vi "Coord window-Initialisation.vi"(6 "Force-clear Listbox":bool, 9 "Coordinate list window refs":T1, 11 "Disable window positioning":bool) -> (0 "error out":errorcluster, 2 "Window size":cluster{"Horisontal":i16, "Vertical":i16}, 3 "VI out":refnum<vi>)   [LabVIEW 2013]
uses:
  Typedefs/Coordinate list window refs.ctl
  Visualisation/Functional Imaging Viewer/SubVIs/Experiment header interface/Typedefs/Save-Load-Save as-Load last enum.ctl
  Globals/Coord window-Globals.vi
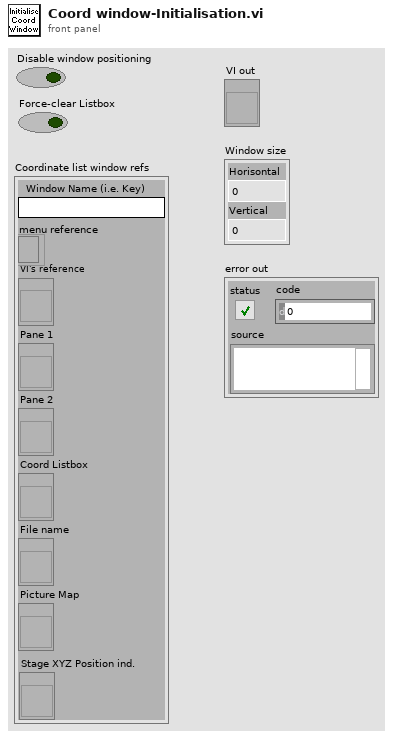
[diagram p1: front panel]
types:
  T1 = typedef "Coordinate list window refs.ctl" = cluster{"Window Name (i.e. Key)":string, "menu reference":refnum<k9>, "VI's reference":refnum<vi>, "Pane 1":refnum<vi>, "Pane 2":refnum<vi>, "Coord Listbox":refnum<vi>, "File name":refnum<vi>, "Picture Map":refnum<vi>, "Stage XYZ Position ind.":refnum<vi>}
  T2 = typedef "Save-Load-Save as-Load last enum.ctl" = enum16{"Save file", "Save file as", "Load file", "Load last file"}
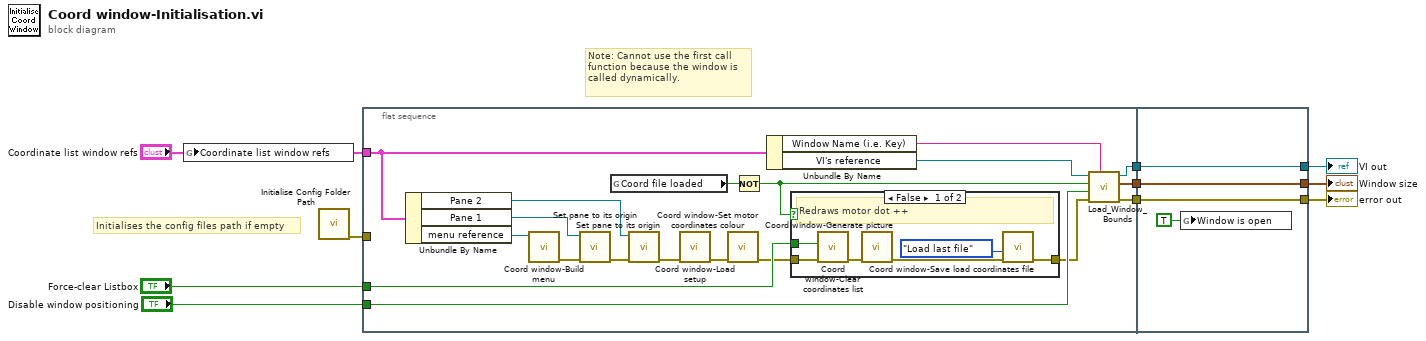
[diagram p0: block diagram]
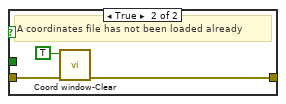
[diagram p2: hidden frame]
diagram:
  # "Initialises the config files path if empty"
  # "Note: Cannot use the first call function because the window is called dynamically."
  n1 = global write "Coord window-Globals.vi" "Coordinate list window refs"("Coordinate list window refs") -> ()
  n2 = call "Initialise Config Folder Path.vi"() -> ("error out"=w1:errorcluster)  [unwired: 9 in, 2 out]
  n3 = flat-sequence {
    tunnel: "Disable window positioning" -> [w24]
    tunnel: "Coordinate list window refs" -> [w19]
    tunnel: [w29] -> w5
    tunnel: [w23] -> w4
    tunnel: [w21] -> w3
    tunnel: "Force-clear Listbox" -> [w15]
    tunnel: w1 -> [_]
    tunnel: [w40] -> w7
    tunnel: [w41] -> w8
    tunnel: [w42] -> w10
    tunnel: w5 -> [w42]
    tunnel: w4 -> [w41]
    tunnel: w3 -> [w40]
    frame #0 {
      n4 = Unbundle By Name(w19) -> ("Pane 2"=w28:refnum<vi>, "Pane 1"=w27:refnum<vi>, "menu reference"=w26:refnum<k9>)
      n5 = call "Coord window-Build menu.vi"("menu"=w26) -> ("error out"=w25:errorcluster)  [unwired: 9 in, 1 out]
      n6 = call "Set pane to its origin.vi"("error in (no error)"=w25, "Pane Reference"=w27) -> ("error out (no error)"=w22:errorcluster)  [unwired: 8 in, 1 out]
      n7 = global read "Coord window-Globals.vi" "Coord file loaded"() -> (w17:bool)
      n8 = call "Set pane to its origin.vi"("error in (no error)"=w22, "Pane Reference"=w28) -> ("error out (no error)"=w14:errorcluster)  [unwired: 8 in, 1 out]
      n9 = call "Coord window-Load setup.vi"("error in (no error)"=w14) -> ("error out"=w13:errorcluster)  [unwired: 10 in]
      n10 = call "Coord window-Set motor coordinates colour.vi"("error in (no error)"=w13) -> ("error out"=w12:errorcluster)  [unwired: 10 in]
      n11 = Not(x=w17) -> (.not. x?=w16:bool)
      n12 = Unbundle By Name(w19) -> ("Window Name (i.e. Key)"=w20:string, "VI's reference"=w18:refnum<vi>)
      n13 = case shown="False" w16 {
        tunnel: w12 -> [w34 w38]
        tunnel: [w30 w37] -> w11
        tunnel: w15 -> [w33 _]
        frame False {
          # "Redraws motor dot ++"
          n14 = call "Coord window-Clear coordinates list.vi"("error in (no error)"=w34, "Enabled? (T)"=w33) -> ("error out"=w35:errorcluster)  [unwired: 9 in]
          n15 = call "Coord window-Generate picture.vi"("error in (no error)"=w35) -> ("error out"=w31:errorcluster)  [unwired: 10 in]
          n16 = call "Coord window-Save load coordinates file.vi"("error in (no error)"=w31, "Function"=Save-Load-Save_as-Load_last_enum."Load last file") -> ("error out"=w30:errorcluster)  [unwired: 9 in]
        }
        frame True {
          # "A coordinates file has not been loaded already"
          n17 = call "Coord window-Clear.vi"("error in (no error)"=w38, "No dialogue"=TRUE) -> ("error out"=w37:errorcluster)  [unwired: 9 in]
        }
      }
      n18 = call "Load_Window_Bounds.vi"("Window Name (i.e. Key)"=w20, "error in"=w11, "Disable"=w24, "First Call"=w16, "Window VI's Ref"=w18) -> ("error out"=w29:errorcluster, "Window size"=w23:cluster{"Horisontal":i16, "Vertical":i16}, "reference out"=w21:refnum<vi>)  [unwired: 3 in, 1 out]
    }
    frame #1 {
      n19 = global write "Coord window-Globals.vi" "Window is open"(TRUE ("Window is open")) -> ()
    }
  }
  "error out" <- w10
  "Window size" <- w8
  "VI out" <- w7
